vi "whiskycola_subvi.vi"() -> (14 "whisk quantity":dbl, 15 "whisky time":dbl, 16 "whisky message":string, 17 "cola quantity":dbl, 18 "cola time":dbl, 19 "cola message":string)   [LabVIEW 2019]
uses:
  <vilib>/Utility/file.llb/Read Delimited Spreadsheet (string).vi
panel:
  out "cola":string
  out "whisky":string
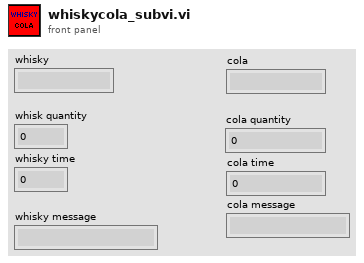
[diagram p1: front panel]
types:
  T1 = cluster{"first row[0]":string, "first row[1]":string, "first row[2]":string, "first row[3]":string, "first row[4]":string, "first row[5]":string, "first row[6]":string, "first row[7]":string, "first row[8]":string}
  T2 = cluster{"Juice":string, "juicequantity":dbl, "juicetime":dbl, "juice message":string}
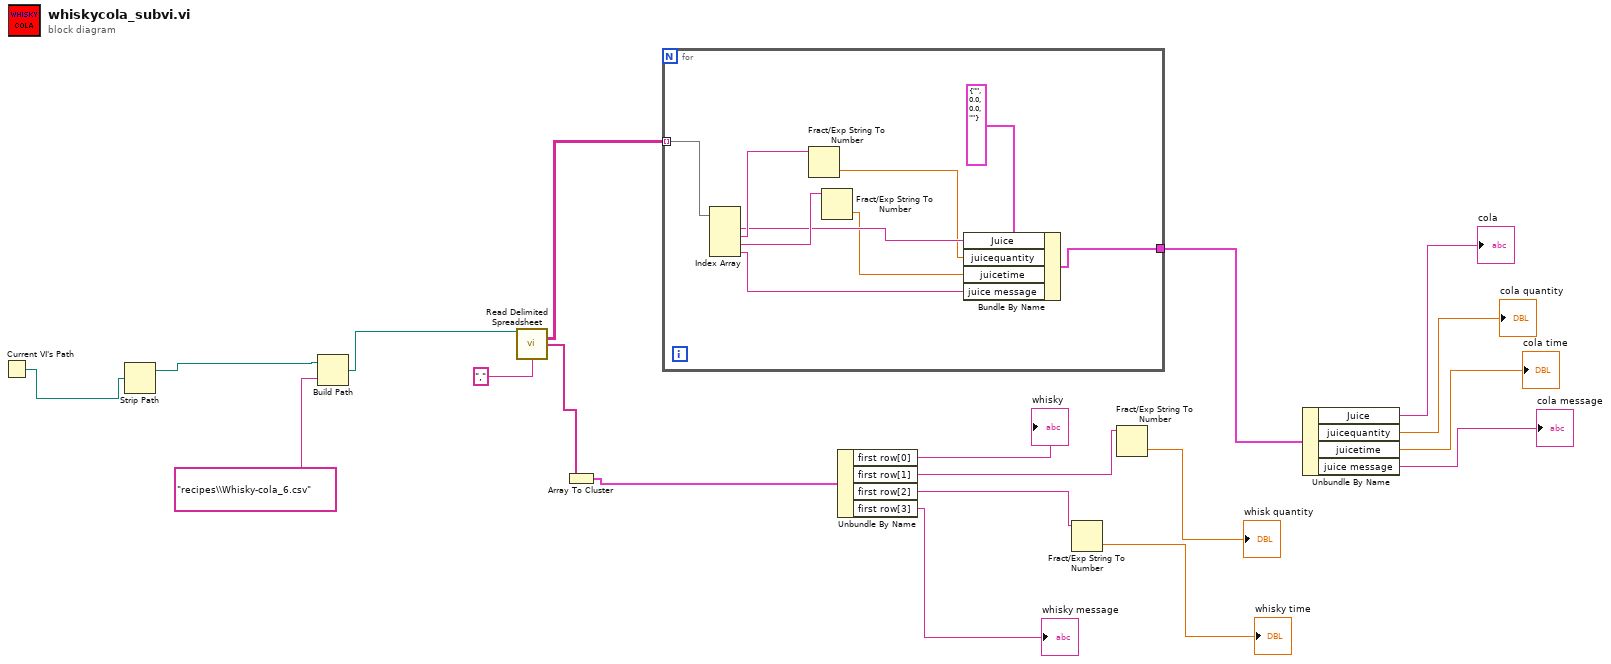
[diagram p0: block diagram]
diagram:
  n1 = Current VI's Path() -> (path=w2:path)
  n2 = Strip Path(path=w2) -> (stripped path=w4:path)  [unwired: 1 out]
  n3 = Build Path(base path=w4, name or relative path="recipes\\Whisky-cola_6.csv") -> (appended path=w1:path)
  n4 = call-poly <vilib>:"Read Delimited Spreadsheet.vi"("file path (dialog if empty)"=w1, "delimiter (\\t)"="," ("delimiter (\\t)")) -> ("all rows"=w18:string[][], "first row"=w17:string[])  [unwired: 8 in, 4 out]
  n5 = Array To Cluster(array=w17) -> (cluster=w16:T1)
  n6 = for {
    tunnel: w18 -> [w28] mode=indexing
    tunnel: [w20] -> w13
    n7 = Index Array(array=w28) -> (element #1=w24:string, element #2=w27:string, element #3=w26:string, element #4=w21:string)  [unwired: 4 in]
    n8 = Fract/Exp String To Number(string=w27) -> (number=w23:dbl)  [unwired: 3 in, 1 out]
    n9 = Fract/Exp String To Number(string=w26) -> (number=w22:dbl)  [unwired: 3 in, 1 out]
    n10 = Bundle By Name(cluster=T2 {"Juice"="", "juicequantity"=0.0, "juicetime"=0.0, "juice message"=""} ("Cluster"), "Juice"=w24, "juicequantity"=w23, "juicetime"=w22, "juice message"=w21) -> (w20:T2)
  }
  n11 = Unbundle By Name(w16) -> ("first row[0]"=→"whisky":string, "first row[1]"=w8:string, "first row[2]"=w6:string, "first row[3]"=→"whisky message":string)
  n12 = Fract/Exp String To Number(string=w6) -> (number=→"whisky time":dbl)  [unwired: 3 in, 1 out]
  n13 = Fract/Exp String To Number(string=w8) -> (number=→"whisk quantity":dbl)  [unwired: 3 in, 1 out]
  n14 = Unbundle By Name(w13) -> ("Juice"=→"cola":string, "juicequantity"=→"cola quantity":dbl, "juicetime"=→"cola time":dbl, "juice message"=→"cola message":string)
